vi "Is Same Task.vi"(9 "Task in 2":refnum<class "Task.lvclass">, 11 "Task in":refnum<class "Task.lvclass">) -> (2 "Same Task?":bool)   [LabVIEW 2017, in "Task Interface.lvlib" / "Task.lvclass"]
uses:
  Task.lvclass
  Task.lvclass/Task.ctl
  Get Name.vi
  Get BuildSpec Name.vi
  Get Target.vi
  Get ProjectName.vi
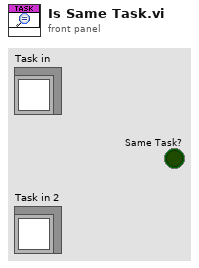
[diagram p1: front panel]
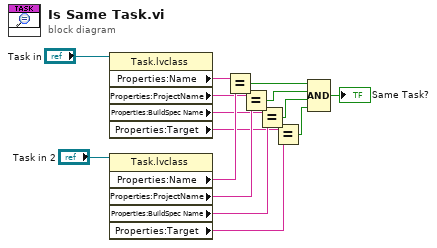
[diagram p0: block diagram]
diagram:
  n1 = property class="Task.lvclass"(reference="Task in") -> ("Properties:Name"=w13:string, "Properties:ProjectName"=w11:string, "Properties:BuildSpec Name"=w9:string, "Properties:Target"=w7:string)  [unwired: 1 in, 2 out]
  n2 = property class="Task.lvclass"(reference="Task in 2") -> ("Properties:Name"=w12:string, "Properties:ProjectName"=w10:string, "Properties:BuildSpec Name"=w8:string, "Properties:Target"=w6:string)  [unwired: 1 in, 2 out]
  n3 = Equal?(x=w13, y=w12) -> (x = y?=w5:bool)
  n4 = Equal?(x=w11, y=w10) -> (x = y?=w4:bool)
  n5 = Equal?(x=w9, y=w8) -> (x = y?=w3:bool)
  n6 = Equal?(x=w7, y=w6) -> (x = y?=w2:bool)
  n7 = Compound Arithmetic op=AND(w5, w4, w3, w2) -> (→"Same Task?":bool)
